vi "Configure_LED_Waveform.vi"   [LabVIEW 2015]
uses:
  <vilib>/Utility/file.llb/Read From Spreadsheet File (DBL).vi
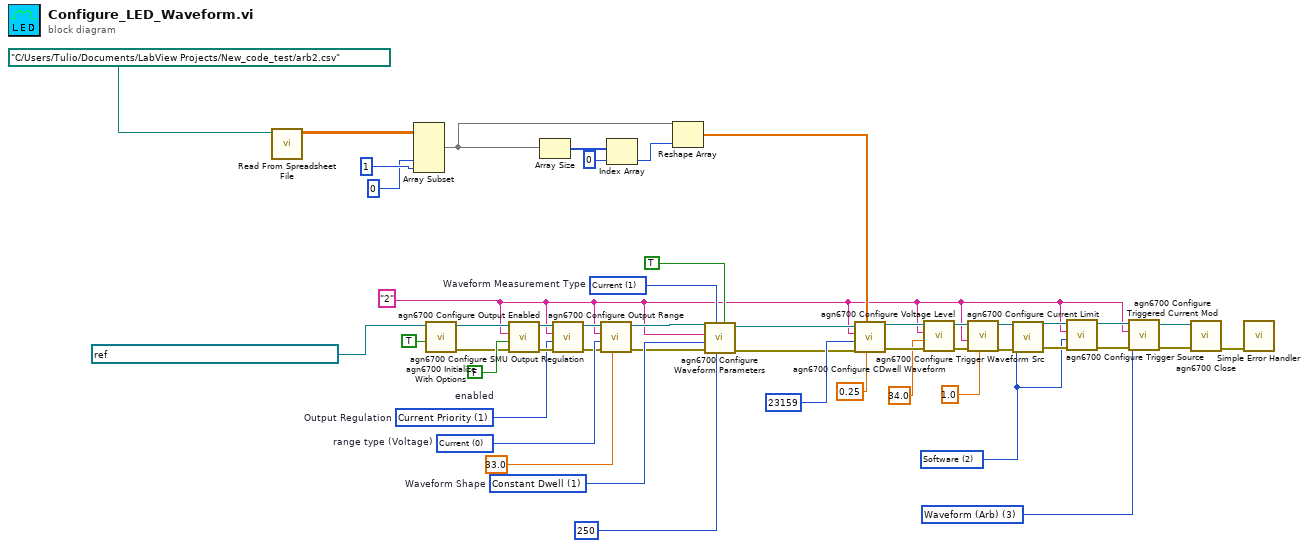
[diagram p0: block diagram]
diagram:
  w9 = 3 items=["Fixed", "Step", "List", "Waveform (Arb)"] ("Current Mode (Fixed)")
  w12 = 2 items=["Immediate", "External", "Software"] ("Waveform Trigger Source (Immediate)")
  w2 = "2" ("channel name (\"\")")
  w45 = FALSE  # enabled
  w33 = 0 items=["Voltage"=1, "Current"=0]  # range type (Voltage)
  w36 = 1 items=["Voltage", "Current"]  # Waveform Measurement Type
  w39 = 1 items=["Voltage Priority", "Current Priority"]  # Output Regulation
  w38 = 1 items=["None", "Constant Dwell", "Exponential", "Pulse", "Ramp", "Sequence", "Sinsuoid", "Staircase", "Step", "Trapezoid", "Undefined"]  # Waveform Shape
  n1 = call-poly <vilib>:"Read From Spreadsheet File.vi"("file path (dialog if empty)"=path "C:/Users/Tulio/Documents/LabView Projects/New_code_test/arb2.csv") -> ("all rows"=w17:dbl[][])  [unwired: 6 in, 4 out]
  n2 = Array Subset "Array Subset"(array=w17, index (col)=0 ("index"), length (col)=1 ("length")) -> (w19:dbl[][])  [unwired: 2 in]
  n3 = call <instrlib>:"agn6700 Initialize With Options.vi"("Reset Device (Yes)"=TRUE, "resource name"=refnum<k15> "USB0::0x0957::0x0F07::MY53002228::INSTR") -> ("error out"=w44:errorcluster, "instrument handle out"=w41:refnum<k15>)  [unwired: 3 in, 5 out]
  n4 = call <instrlib>:"agn6700 Configure Output Enabled.vi"("error in (no error)"=w44, "Enabled (True)"=w45, "Channel Name (\"\")"=w2, "instrument handle"=w41) -> ("error out"=w43:errorcluster, "instrument handle out"=w42:refnum<k15>)  [unwired: 6 out]
  n5 = Array Size(array=w19) -> (size(s)=w20:i32[])
  n6 = call <instrlib>:"agn6700 Configure SMU Output Regulation.vi"("error in (no error)"=w43, "Output Regulation (Voltage Priority)"=w39, "Channel Name (\"\")"=w2, "instrument handle"=w42) -> ("error out"=w31:errorcluster, "instrument handle out"=w30:refnum<k15>)  [unwired: 6 out]
  n7 = call <instrlib>:"agn6700 Configure Output Range.vi"("Range (0.02)"=33.0 ("range (0.02)"), "error in (no error)"=w31, "Range Type (Voltage)"=w33, "Channel Name (\"\")"=w2, "instrument handle"=w30) -> ("error out"=w28:errorcluster, "instrument handle out"=w29:refnum<k15>)  [unwired: 5 out]
  n8 = Index Array "Index Array"(array=w20, index=0) -> (element=w22:i32)
  n9 = Reshape Array "Reshape Array"(w19, w22) -> (w15:dbl[])
  n10 = call <instrlib>:"agn6700 Configure Waveform Parameters.vi"("Enable Waveform Termination (Off)"=TRUE, "Waveform Count (1)"=250, "Waveform Measurement Type (Voltage)"=w36, "error in (no error)"=w28, "Waveform Shape (None)"=w38, "Channel Name (\"\")"=w2, "instrument handle"=w29) -> ("error out"=w47:errorcluster, "instrument handle out"=w46:refnum<k15>)  [unwired: 3 out]
  n11 = call <instrlib>:"agn6700 Configure CDwell Waveform.vi"("Constant Dwell Time (0.001)"=0.25, "Constant Dwell Level"=w15, "error in (no error)"=w47, "Constant Dwell Level Wfm Size"=23159, "Channel Name (\"\")"=w2, "instrument handle"=w46) -> ("error out"=w26:errorcluster, "instrument handle out"=w27:refnum<k15>)  [unwired: 4 in]
  n12 = call <instrlib>:"agn6700 Configure Voltage Level.vi"("error in (no error)"=w26, "Level (0.02)"=34.0, "Channel Name (\"\")"=w2, "instrument handle"=w27) -> ("error out"=w6:errorcluster, "instrument handle out"=w5:refnum<k15>)  [unwired: 6 in]
  n13 = call <instrlib>:"agn6700 Configure Current Limit.vi"("Limit (0.01)"=1.0, "error in (no error)"=w6, "Channel Name (\"\")"=w2, "instrument handle"=w5) -> ("error out"=w3:errorcluster, "instrument handle out"=w4:refnum<k15>)  [unwired: 6 in]
  n14 = call <instrlib>:"agn6700 Configure Trigger Waveform Src.vi"("error in (no error)"=w3, "Waveform Trigger Source (Immediate)"=w12, "instrument handle"=w4) -> ("error out"=w13:errorcluster, "instrument handle out"=w14:refnum<k15>)  [unwired: 7 in]
  n15 = call <instrlib>:"agn6700 Configure Trigger Source.vi"("error in (no error)"=w13, "Source (Software)"=w12, "Channel Name (\"\")"=w2, "instrument handle"=w14) -> ("error out"=w10:errorcluster, "instrument handle out"=w11:refnum<k15>)  [unwired: 6 in]
  n16 = call <instrlib>:"agn6700 Configure Triggered Current Mod.vi"("error in (no error)"=w10, "Current Mode (Fixed)"=w9, "Channel Name (\"\")"=w2, "instrument handle"=w11) -> ("error out"=w8:errorcluster, "instrument handle out"=w7:refnum<k15>)  [unwired: 6 in]
  n17 = call <instrlib>:"agn6700 Close.vi"("error in (no error)"=w8, "instrument handle"=w7) -> ("error out"=w40:errorcluster)  [unwired: 9 out]
  n18 = call <vilib>:"Simple Error Handler.vi"("error in (no error)"=w40) -> ()  [unwired: 1 in, 8 out]
